vi "String Search If Contain.vi"(10 "String like":string, 11 "Array - String":string[](array[string])) -> (2 "contain array thisString somewhere":bool, 3 "items indexes[]":i32[](array[numeric]))   [LabVIEW 2018]
doc: "Looking inside each String[] item if it contains \"String like\" input value."
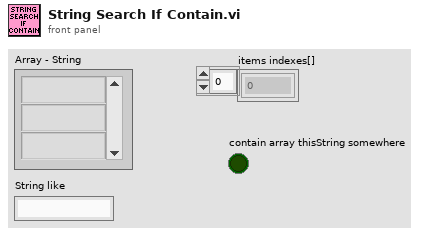
[diagram p1: front panel]
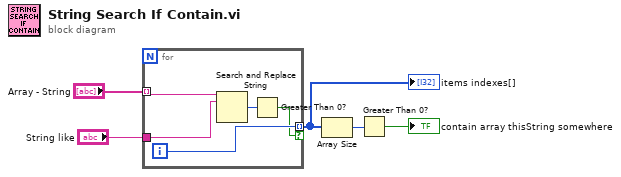
[diagram p0: block diagram]
diagram:
  n1 = for {
    tunnel: "Array - String" -> [w10] mode=indexing
    tunnel: "String like" -> [w9]
    tunnel: [w7] -> w3 mode=indexing if=w6
    i -> [w7]
    n2 = Search and Replace String(input string=w10, search string=w9) -> (number of replacements=w8:i32)  [unwired: 6 in, 3 out]
    n3 = Greater Than 0?(x=w8) -> (x > 0?=w6:bool)
  }
  "items indexes[]" <- w3
  n4 = Array Size(array=w3) -> (size(s)=w2:i32)
  n5 = Greater Than 0?(x=w2) -> (x > 0?=→"contain array thisString somewhere":bool)
